vi "Recall Bar Sample Hall Results.vi"() -> (2 "Bar Sample Hall Results":cluster{"n/p":dbl, "uH":dbl})   [LabVIEW 2016, in "Hall Effect Library.lvlib"]
uses:
  Hall Effect Library.lvlib
  Private/Global Variables/Hall Effect Data.vi
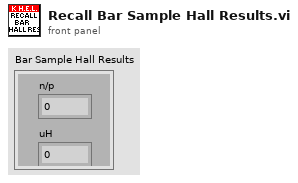
[diagram p1: front panel]
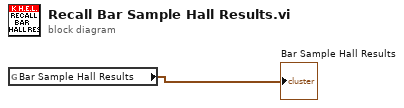
[diagram p0: block diagram]
diagram:
  n1 = global read "Hall Effect Data.vi" "Bar Sample Hall Results"() -> (→"Bar Sample Hall Results":cluster{"n/p":dbl, "uH":dbl})
